vi "NIGoHome.vi"(2 "error in (no error)":errorcluster, 3 "# Axis":i8=1, 4 "Board ID":u8=1 min=1 max=32 step=1) -> (0 "error out":errorcluster, 1 "Bd ID Out":u8)   [LabVIEW 2022 SP3]
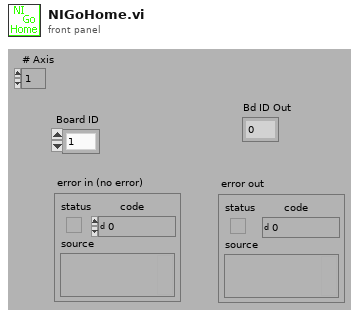
[diagram p1: front panel]
types:
  T1 = enum16{"Absolute Position", "Relative Position", "Velocity", "Relative to Cap Pos", "Modulus Position", "Absolute Contouring", "Relative Contouring"}
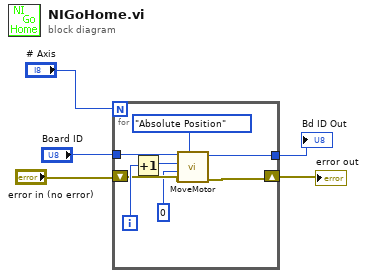
[diagram p0: block diagram]
diagram:
  n1 = for {
    N: "# Axis" -> [_]
    shift-right: [w9] -> w5
    shift-left: "error in (no error)" -> [w10]
    tunnel: [w8] -> w2
    tunnel: "Board ID" -> [w12]
    i -> [w13]
    n2 = Increment(x=w13) -> (x+1=w7:i32)
    n3 = call "MoveMotor.vi"("Position Mode (Absolute)"=T1."Absolute Position", "error in (no error)"=w10, "Target Position (0)"=0, "Axis or Vector Space"=w7, "Motion Bd ID"=w12) -> ("error out"=w9:errorcluster, "Bd ID Out"=w8:u8)  [unwired: 4 in, 1 out]
  }
  "error out" <- w5
  "Bd ID Out" <- w2
